vi "MainGUI.vi"(0 "reference in":refnum<class "MasterGUI.lvclass">, 5 "Error In":errorcluster) -> (14 "reference out":refnum<class "MasterGUI.lvclass">, 19 "Error Out":errorcluster)   [LabVIEW 2021, in "MasterGUI.lvclass"]
doc: "This template is based off of the Queued Message Handler design pattern and the Queued Message Handler project template that ships with LabVIEW.\n\nThe main difference is that the queue is private to this module and communication between modules is performed via Broadcast and Request events.\n\nRequest events are wrapped in public API methods and are handled in the Event Handling Loop (EHL) of this VI. Any module can register for Broadcast events sent by this module. The EHL generates messages based on user interface actions.\n\nThe Message Handling Loop (MHL) processes messages generated by the EHL, or by other messages. The messages are string values, so new messages can be added easily to the Message Cases case structure in the MHL. Each message cluster can also provide an optional value for Message Data, which is a variant that can be converted to whatever message-specific data is required.\n_____\nBased on Delacor QMH Project Template 4.2.0.63.\n\n<b>Note:</b> This VI was modified by the <b>Validate DQMH Module</b> tool to have the module name be passed as the Additional Information parameter with an Error Reported broadcast.\n\n<b>Note:</b> This VI was modified by the <b>Validate DQMH Module</b> tool to call the Release Message Queue VI in the top-level Error case."
uses:
  MasterGUI.lvclass
  MasterGUI_MessageData.ctl
  MasterGUI.lvclass/MasterGUI.ctl
panel:
  out "Last Command":string
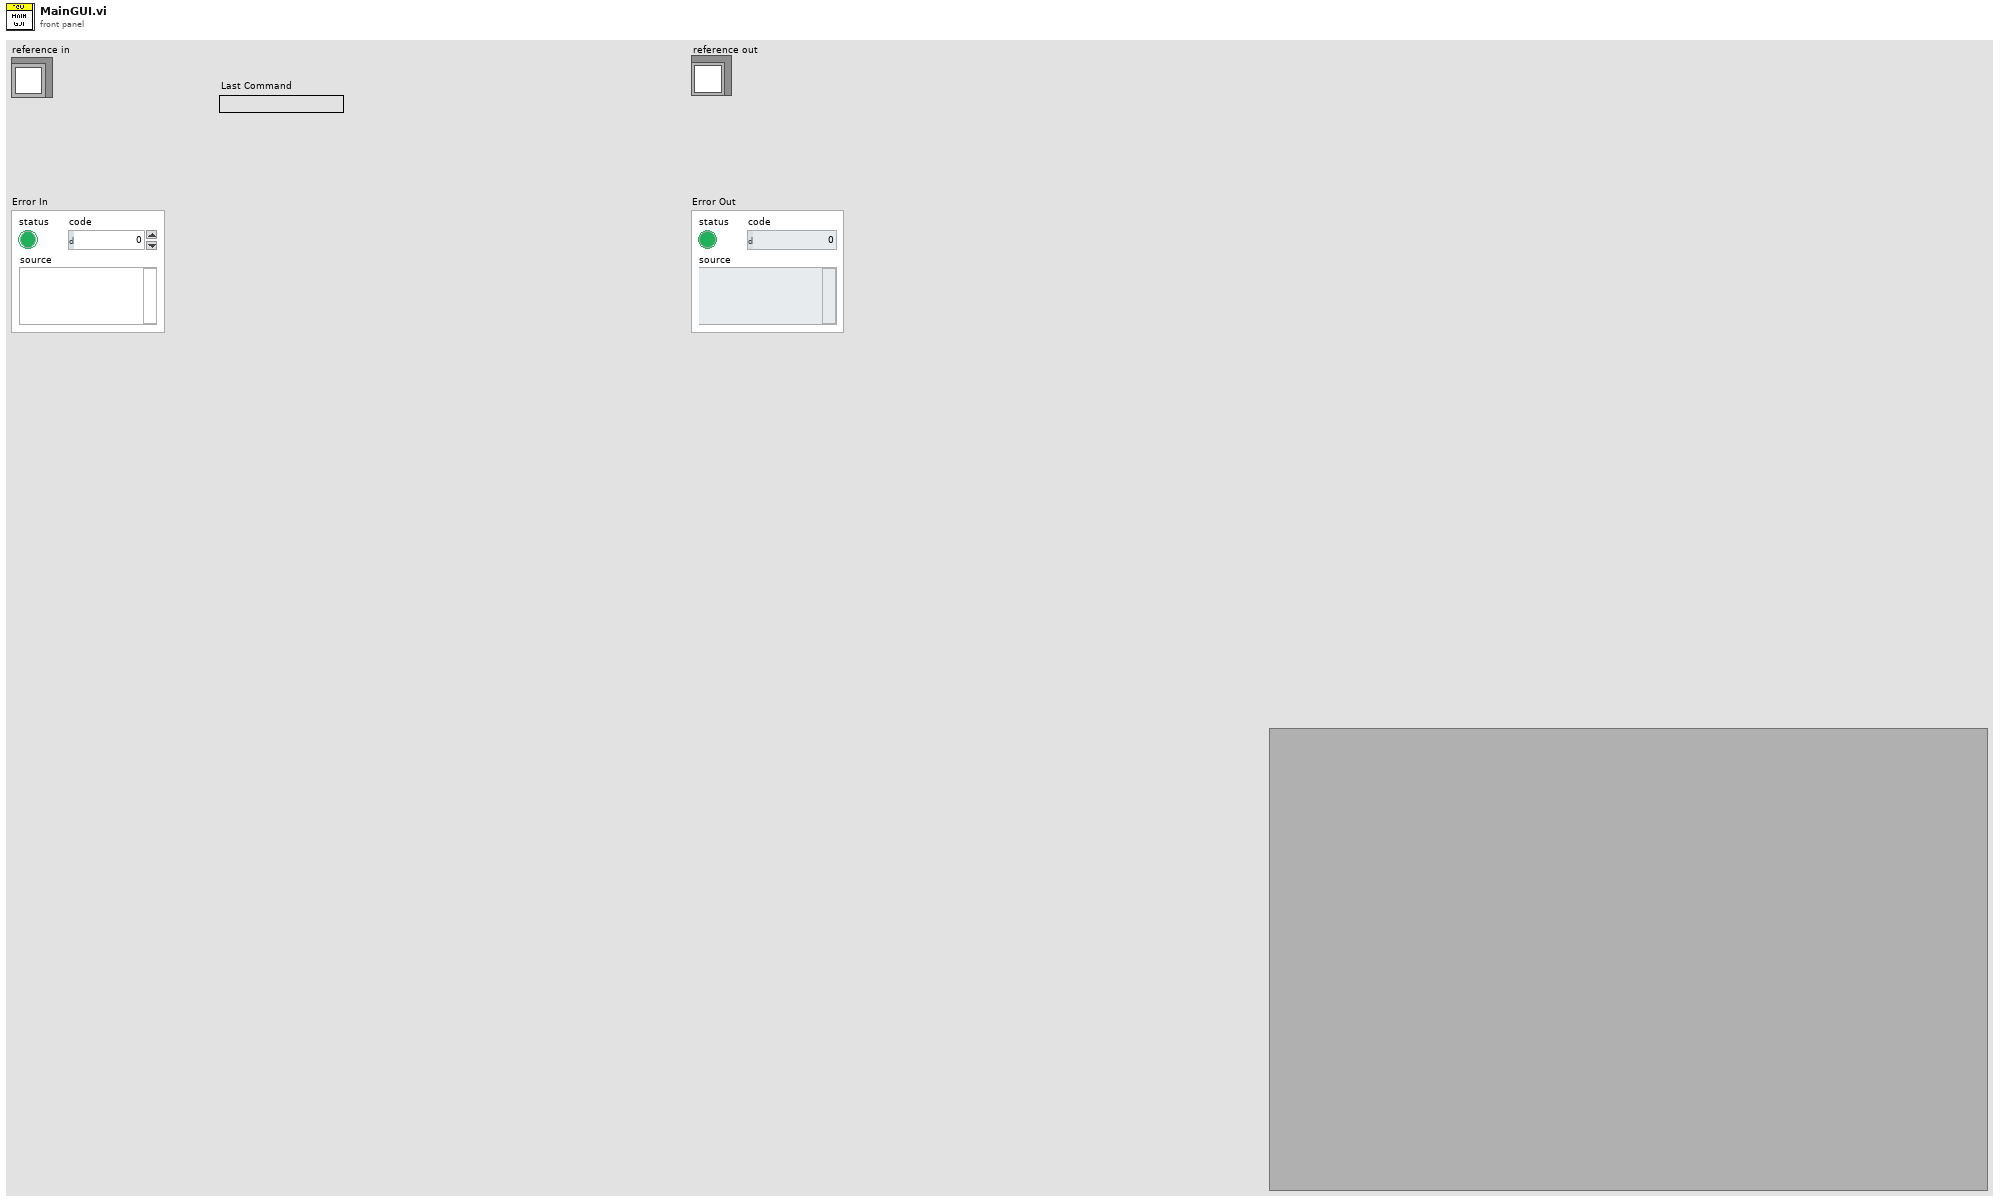
[diagram p1: front panel]
types:
  T1 = typedef "MasterGUI.lvclass/MasterGUI_MessageData.ctl" = cluster{"ShowWindow":cluster{"Send":cluster{"Show":bool}, "Receive":cluster{"Dummy":bool}}}
  T2 = cluster{"Event":refnum<event-registration>, "Command":string, "MessageData":T1, "ReplyQueue":refnum<queue>}
  T3 = cluster{"ReplyQueue":refnum<queue>, "Data":variant}
  T4 = typedef "MasterGUI.lvclass/WindowsProperties.ctl" = cluster{"WindowsTitle":string, "Centered":bool, "Minimizable":bool, "Resizable":bool, "State":enum32{"Invalid", "Standard", "Closed", "Hidden", "Minimized", "Maximized"}, "Position":cluster{"X":i32, "Y":i32}, "Size":cluster{"X":i32, "Y":i32}}
  T5 = enum32{"Invalid", "Standard", "Closed", "Hidden", "Minimized", "Maximized"}
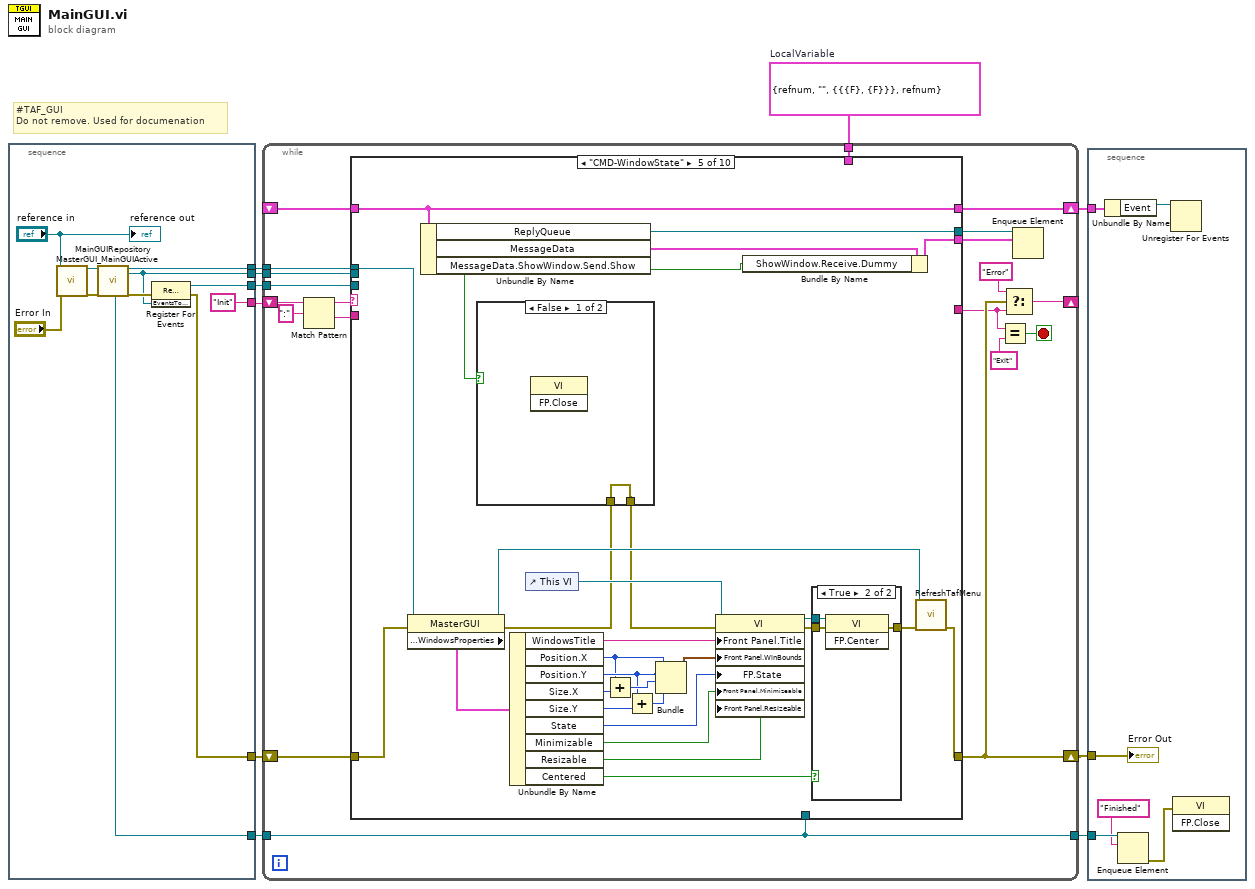
[diagram p0: block diagram]
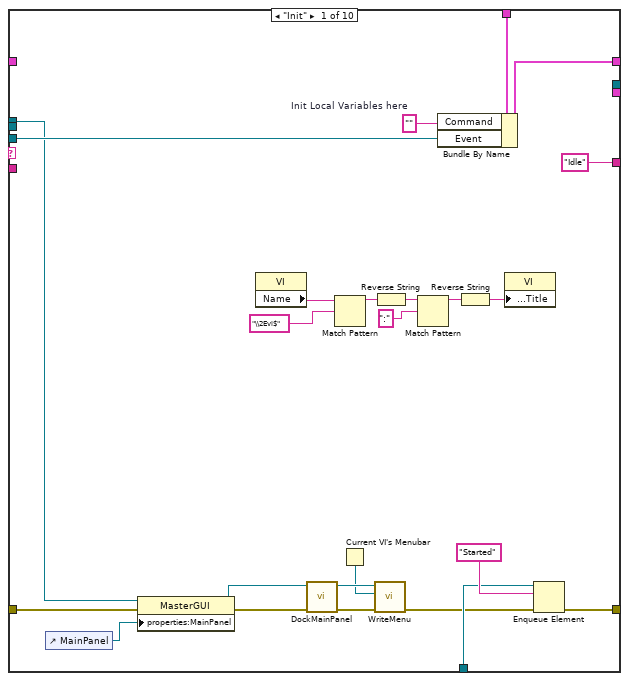
[diagram p2: hidden frame]
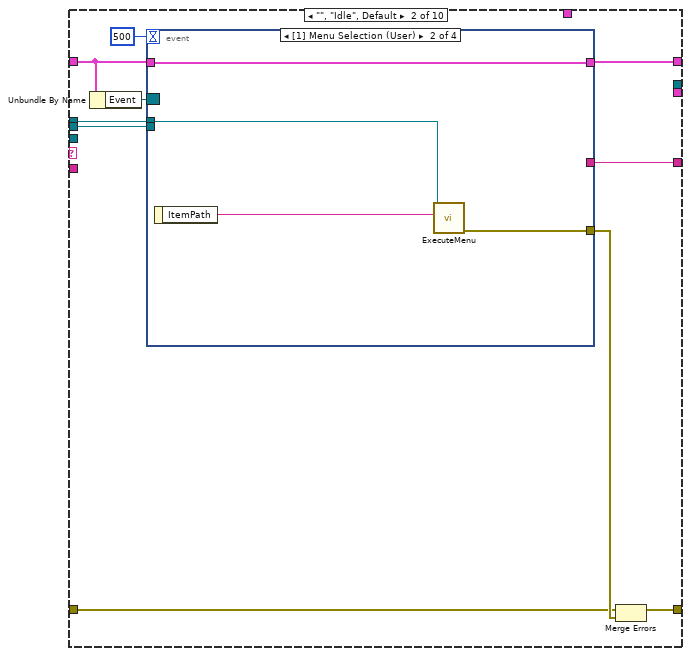
[diagram p3: hidden frame]
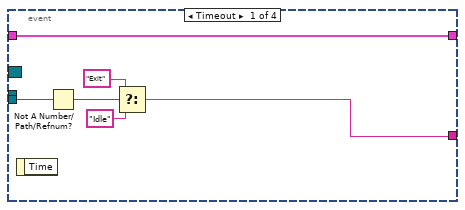
[diagram p4: hidden frame]
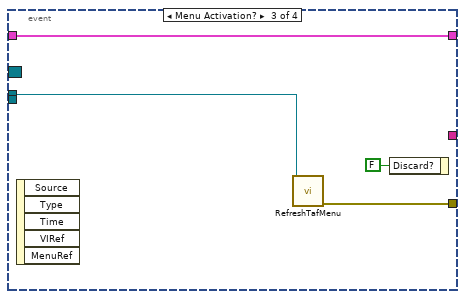
[diagram p5: hidden frame]
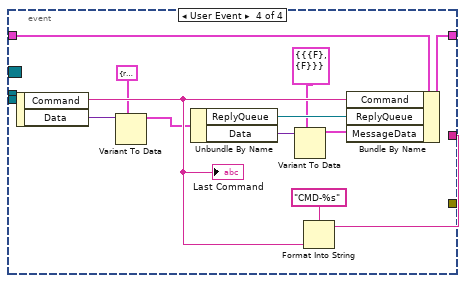
[diagram p6: hidden frame]
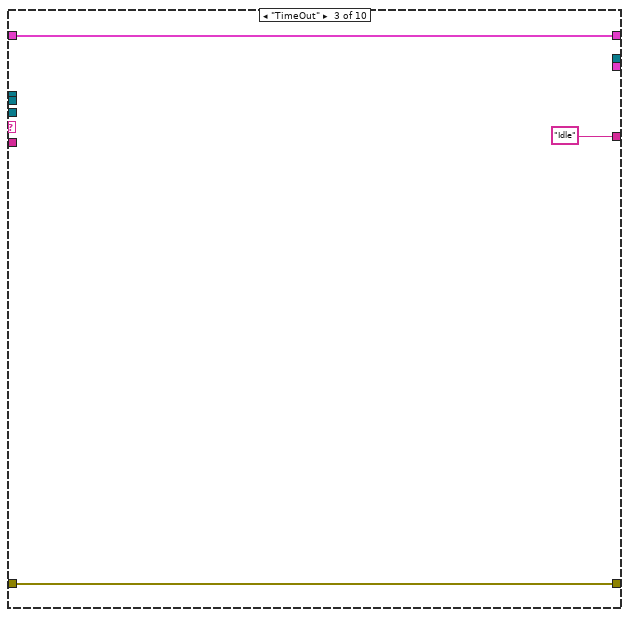
[diagram p7: hidden frame]
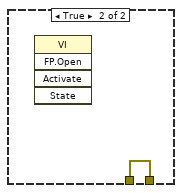
[diagram p10: hidden frame]
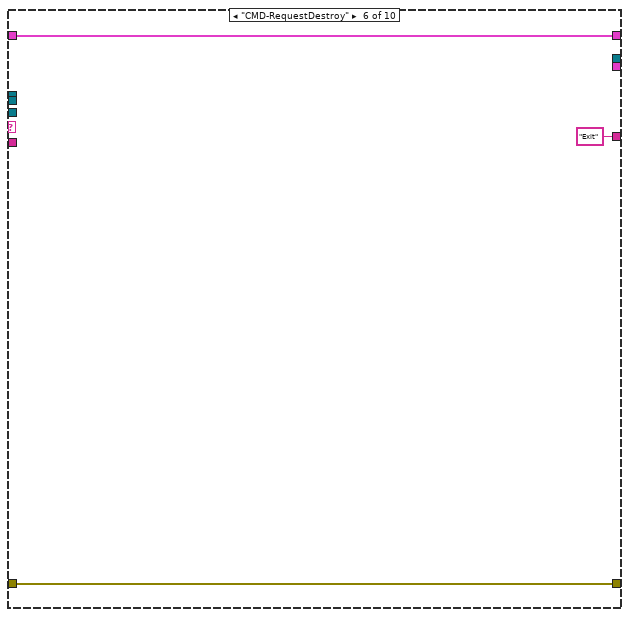
[diagram p11: hidden frame]
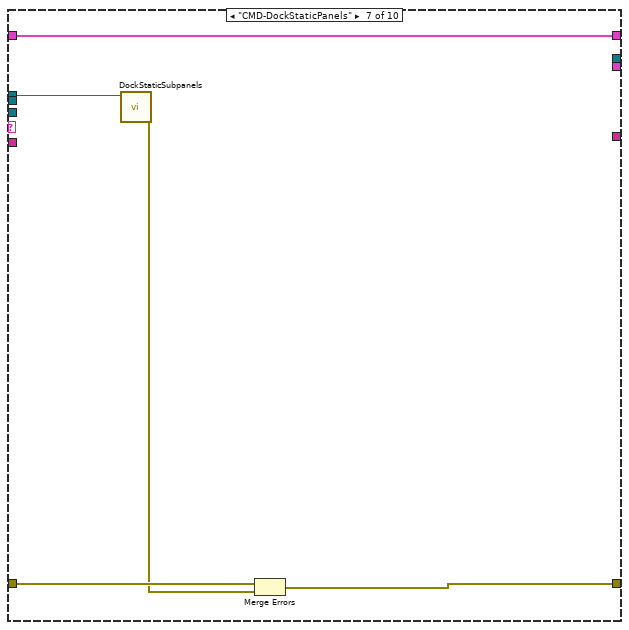
[diagram p12: hidden frame]
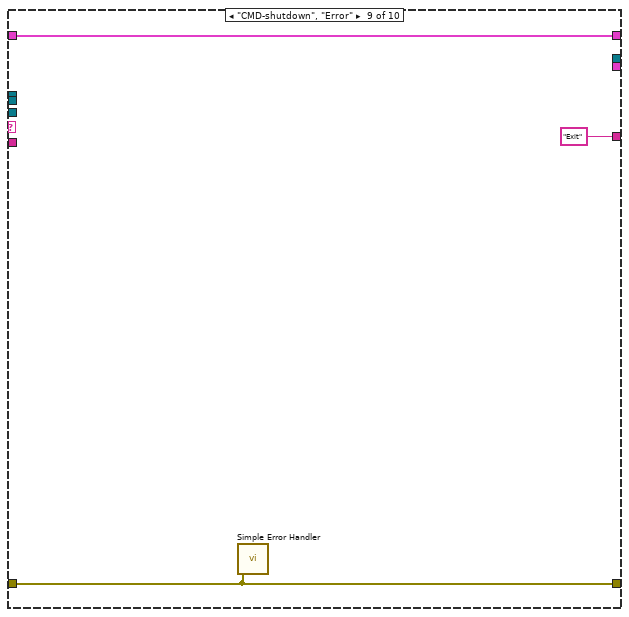
[diagram p14: hidden frame]
diagram:
  w5 = T2 {"Event"=refnum, "Command"="", "MessageData"={"ShowWindow"={"Send"={"Show"=FALSE}, "Receive"={"Dummy"=FALSE}}}, "ReplyQueue"=refnum}  # LocalVariable
  # "#TAF_GUI\nDo not remove. Used for documenation"
  n1 = stacked-sequence {
    tunnel: [w17] -> w10
    tunnel: [w21] -> w8
    tunnel: [w15] -> w7
    tunnel: ["Init"] -> w6
    tunnel: [w18] -> w3
    tunnel: [w16] -> w1
    frame #0 {
      n2 = call "MasterGUI_MainGUIActive.vi"("ErrorIn"="Error In", "ReferenceIn"="reference in") -> ("ErrorOut"=w11:errorcluster, "ReferenceIn"=w13:refnum<class "MasterGUI.lvclass">)  [unwired: 8 in]
      n3 = call "MainGUIRepository.vi"("ReferenceIn"=w13, "ErrorIn"=w11) -> ("ProcessSyncQueue"=w18:refnum<queue>, "ReferenceOut"=w21:refnum<class "MasterGUI.lvclass">, "EventsToProcess"=w16:refnum<user-event>, "ErrorOut"=w19:errorcluster)  [unwired: 10 in, 4 out]
      n4 = register-events(error in=w19, w16) -> (reference out=w15:refnum<event-registration>, error out=w17:errorcluster)  [unwired: 1 in]
      "reference out" <- "reference in"
    }
  }
  n5 = while {
    shift-right: [w34] -> w9
    shift-left: w10 -> [w39]
    tunnel: w8 -> [w40]
    tunnel: w7 -> [w41]
    shift-right: [w32] -> _
    shift-left: w6 -> [w37]
    shift-right: [w28] -> w4
    shift-left: _ -> [w27]
    tunnel: w5 -> [w26]
    tunnel: [w23] -> w2
    tunnel: w3 -> [w23]
    tunnel: w1 -> [w22]
    stop <- w29 stop-if-true
    n6 = Match Pattern(string=w37, regular expression=":") -> (before substring=w36:string, after substring=w35:string)  [unwired: 1 in, 2 out]
    n7 = case shown="\"CMD-WindowState\"" w36 {
      tunnel: w39 -> [w50 w66 w104 w106 w128 w143 w148 w150 w151 w155]
      tunnel: [w52 w68 w104 w106 w109 w143 w145 w150 w151 w155] -> w34
      tunnel: w41 -> [w54 _ _ _ _ _ _ _ _ _]
      tunnel: w40 -> [w49 w70 _ _ w129 _ w146 _ _ _]
      tunnel: w35 -> [_ _ _ _ _ _ _ _ _ _]
      tunnel: ["Idle" ("t") w75 "Idle" ("t") _ _ "Exit" ("y") _ _ "Exit" ("y") _] -> w31
      tunnel: [w65 w74 w102 w105 w134 w142 w147 w149 w152 w154] -> w28
      tunnel: w27 -> [_ w73 w102 w105 w134 w142 w147 w149 w152 w154]
      tunnel: w26 -> [w62 _ _ _ _ _ _ _ _ _]
      tunnel: [_ _ _ _ w133 _ _ _ _ _] -> w25
      tunnel: [_ _ _ _ w131 _ _ _ _ _] -> w24
      tunnel: w23 -> [w51 _ _ _ _ _ _ _ _ _]
      tunnel: w22 -> [_ w69 _ _ _ _ _ _ _ _]
      frame "Init" {
        w64 = ""  # Init Local Variables here
        n8 = control-ref of="MainPanel"() -> (w48:refnum<vi>)
        n9 = property class="MasterGUI"(reference=w49, error in=w50, "properties:MainPanel"=w48) -> (reference out=w47:refnum<class "MasterGUI.lvclass">, error out=w46:errorcluster)
        n10 = property class="VI"() -> ("Name"=w61:string)  [unwired: 2 in, 2 out]
        n11 = call-dynamic "DockMainPanel.vi"("ErrorIn"=w46, "ReferenceIn"=w47) -> ("ErrorOut"=w45:errorcluster, "ReferenceIn"=w44:refnum<class "MasterGUI.lvclass">)  [unwired: 8 in]
        n12 = Match Pattern(string=w61, regular expression="\\2Evi$") -> (before substring=w59:string)  [unwired: 1 in, 3 out]
        n13 = Current VI's Menubar() -> (w42:refnum<k9>)
        n14 = call-dynamic "WriteMenu.vi"("ErrorIn"=w45, "Menu"=w42, "ReferenceIn"=w44) -> ("ErrorOut"=w43:errorcluster)  [unwired: 7 in, 1 out]
        n15 = Reverse String(1:w59) -> (0:w58:string)
        n16 = Match Pattern(string=w58, regular expression=":") -> (before substring=w56:string)  [unwired: 1 in, 3 out]
        n17 = Bundle By Name(cluster=w62, "Command"=w64, "Event"=w54) -> (w65:T2)
        n18 = Reverse String(1:w56) -> (0:w55:string)
        n19 = property class="VI"("Front Panel.Title"=w55) -> ()  [unwired: 2 in, 2 out]
        n20 = Enqueue Element(queue=w51, element="Started", error in (no error)=w43) -> (error out=w52:errorcluster)  [unwired: 1 in, 2 out]
      }
      frame "", "Idle", Default {
        n21 = Unbundle By Name(w73) -> ("Event"=w72:refnum<event-registration>)
        n22 = event shown="[1] Menu Selection (User)" {
          selector: w72 -> [_ _ _ _]
          dyn-events: _ -> [_ _ _ _]
          timeout: 500 -> [_ _ _ _]
          tunnel: [w78 _ _ w98] -> w75
          tunnel: w73 -> [w81 w85 w89 w101]
          tunnel: [w81 w85 w89 w100] -> w74
          tunnel: w70 -> [_ w82 w86 _]
          tunnel: w69 -> [w77 _ _ _]
          tunnel: [_ w83 w87 _] -> w67
          event Timeout {
            n23 = event-data() -> ()  [unwired: 1 in, 1 out]
            n24 = Not A Number/Path/Refnum?(number/path/refnum=w77) -> (NaN/Path/Refnum?=w76:bool)
            n25 = Select(t="Exit", s=w76, f="Idle" ("t")) -> (s? t:f=w78:string)
          }
          event Menu Selection (User) {
            n26 = event-data() -> ("ItemPath"=w84:string)  [unwired: 1 in]
            n27 = call-dynamic "ExecuteMenu.vi"("ItemPath"=w84, "MasterGUIIn"=w82) -> ("ErrorOut"=w83:errorcluster)  [unwired: 8 in, 1 out]
          }
          event Menu Activation? {
            n28 = event-data() -> ()  [unwired: 1 in, 5 out]
            n29 = call-dynamic "RefreshTafMenu.vi"("ObjectIn"=w86) -> ("ErrorOut"=w87:errorcluster)  [unwired: 9 in, 1 out]
            n30 = event-data("Discard?"=FALSE) -> ()  [unwired: 1 in, 1 out]
          }
          event User Event {
            n31 = event-data() -> ("Command"=w97:string, "Data"=w96:variant)  [unwired: 1 in]
            "Last Command" <- w97
            n32 = Variant To Data(type=T3 {"ReplyQueue"=refnum, "Data"=variant} ("output cluster"), Variant=w96) -> (data=w94:T3)  [unwired: 1 in, 1 out]
            n33 = Unbundle By Name(w94) -> ("ReplyQueue"=w93:refnum<queue>, "Data"=w92:variant)
            n34 = Variant To Data(type=T1 {"ShowWindow"={"Send"={"Show"=FALSE}, "Receive"={"Dummy"=FALSE}}} ("MessageData"), Variant=w92) -> (data=w91:T1)  [unwired: 1 in, 1 out]
            n35 = Format Into String(format string="CMD-%s", w97) -> (resulting string=w98:string)  [unwired: 2 in, 1 out]
            n36 = Bundle By Name(cluster=w101, "Command"=w97, "ReplyQueue"=w93, "MessageData"=w91) -> (w100:T2)
          }
        }
        n37 = Merge Errors(w66, w67) -> (w68:errorcluster)
      }
      frame "TimeOut" {
      }
      frame "---- COMMANDS START----" {
      }
      frame "CMD-WindowState" {
        n38 = property class="MasterGUI"(reference=w129, error in=w128) -> (reference out=w125:refnum<class "MasterGUI.lvclass">, error out=w108:errorcluster, "properties:WindowsProperties"=w124:T4)
        n39 = Unbundle By Name(w134) -> ("ReplyQueue"=w133:refnum<queue>, "MessageData"=w132:T1, "MessageData.ShowWindow.Send.Show"=w130:bool)
        n40 = case shown="False" w130 {
          tunnel: [w139 w140] -> w107
          tunnel: w108 -> [w139 w140]
          frame False {
            n41 = invoke class="VI" method="FP.Close"() -> ()  [unwired: 3 in, 3 out]
          }
          frame True {
            n42 = invoke class="VI" method="FP.Open"() -> ()  [unwired: 5 in, 5 out]
          }
        }
        n43 = Unbundle By Name(w124) -> ("WindowsTitle"=w123:string, "Position.X"=w117:i32, "Position.Y"=w118:i32, "Size.X"=w122:i32, "Size.Y"=w121:i32, "State"=w112:T5, "Minimizable"=w111:bool, "Resizable"=w110:bool, "Centered"=w113:bool)
        n44 = control-ref of="This VI"() -> (w127:refnum<vi>)
        n45 = Add(x=w117, y=w122) -> (x+y=w119:i32)
        n46 = Add(x=w118, y=w121) -> (x+y=w120:i32)
        n47 = Bundle("X"=w117, "Y"=w118, w119, w120) -> (w116:cluster{"X":i32, "Y":i32, i32, i32})  [unwired: 1 in]
        n48 = property class="VI"(reference=w127, error in=w107, "Front Panel.Title"=w123, "Front Panel.WinBounds"=w116, "FP.State"=w112, "Front Panel.Minimizeable"=w111, "Front Panel.Resizeable"=w110) -> (reference out=w114:refnum<vi>, error out=w126:errorcluster)
        n49 = Bundle By Name(cluster=w132, "ShowWindow.Receive.Dummy"=w130) -> (w131:T1)
        n50 = case shown="True" w113 {
          tunnel: w126 -> [w135 w138]
          tunnel: [w135 w137] -> w115
          tunnel: w114 -> [_ w136]
          frame False {
          }
          frame True {
            n51 = invoke class="VI" method="FP.Center"(reference=w136, error in=w138) -> (error out=w137:errorcluster)  [unwired: 1 in, 2 out]
          }
        }
        n52 = call-dynamic "RefreshTafMenu.vi"("ErrorIn"=w115, "ObjectIn"=w125) -> ("ErrorOut"=w109:errorcluster)  [unwired: 8 in, 1 out]
      }
      frame "CMD-RequestDestroy" {
      }
      frame "CMD-DockStaticPanels" {
        n53 = call-dynamic "DockStaticSubpanels.vi"("ReferenceIn"=w146) -> ("ErrorOut"=w144:errorcluster)  [unwired: 9 in, 1 out]
        n54 = Merge Errors(w148, w144) -> (w145:errorcluster)
      }
      frame "----- COMMANDS END ----" {
      }
      frame "CMD-shutdown", "Error" {
        n55 = call <vilib>:"Simple Error Handler.vi"("error in (no error)"=w151) -> ()  [unwired: 4 in, 5 out]
      }
      frame "----- UI ACTIONS -----" {
      }
    }
    n56 = Equal?(x=w31, y="Exit") -> (x = y?=w29:bool)
    n57 = Select(t="Error", s=w34, f=w31) -> (s? t:f=w32:string)
    n58 = Enqueue Element(queue=w25, element=w24) -> ()  [unwired: 2 in, 3 out]
  }
  n59 = stacked-sequence {
    tunnel: w9 -> [w161]
    tunnel: w2 -> [w158]
    tunnel: w4 -> [w160]
    frame #0 {
      n60 = Unbundle By Name(w160) -> ("Event"=w159:refnum<event-registration>)
      n61 = Enqueue Element(queue=w158, element="Finished") -> (error out=w157:errorcluster)  [unwired: 2 in, 2 out]
      n62 = Unregister For Events(event registration refnum=w159) -> ()  [unwired: 1 in, 1 out]
      n63 = invoke class="VI" method="FP.Close"(error in=w157) -> ()  [unwired: 2 in, 3 out]
      "Error Out" <- w161
    }
  }
